vi "PYTHON Get Version and Types__ogtk.vi"(4 "error in (no error)":errorcluster) -> (0 "error out":errorcluster, 2 "types":string[](array[string]), 3 "script server version":string)   [LabVIEW 2012]
doc: "This function returns a version string indicating the Python version implemented in the Python shared library server, (Date and Time when the shared library was created), and [the compiler used to create that shared library]."
uses:
  <userlib>/_OpenG.lib/labpython/lvpython.dll
panel:
  # "PYTHON Get Version and Types.vi\n\nRetrieve the Python shared library version and the supported types\n\nCopyright (C) 2002 Rolf Kalbermatter rolf.kalbermatter@citeng.com\nCopyright (C) 2002 James Kring jim@jimkring.com\n\nPlease visit http://www.OpenG.org to learn about the\nOpen Source LabVIEW software movement.\n\nThis library is free software; you can redistribute it and/or\nmodify it under the terms of the GNU Lesser General Public\nLicense as published by the Free Software Foundation; either\nversion 2.1 of the License, or (at your option) any later version.\nThis library is distributed in the hope that it will be useful,\nbut WITHOUT ANY WARRANTY; without even the implied warranty of\nMERCHANTABILITY or FITNESS FOR A PARTICULAR PURPOSE. See the GNU\nLesser General Public License for more details.\nYou should have received a copy of the GNU Lesser General Public\nLicense along with this library; if not, write to the Free Software\nFoundation, Inc., 59 Temple Place, Suite 330, Boston, MA 02111-1307 USA"
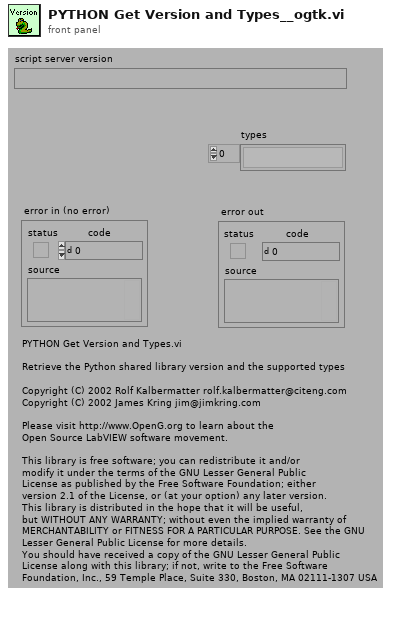
[diagram p1: front panel]
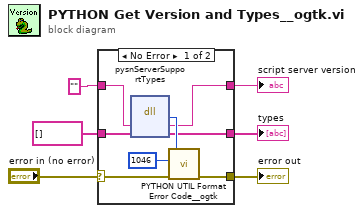
[diagram p0: block diagram]
diagram:
  n1 = case shown="No Error" "error in (no error)" {
    selector: "error in (no error)" -> [w13 w17]
    tunnel: [w10 w15] -> w6
    tunnel: [w12 w17] -> w4
    tunnel: [w9 w16] -> w3
    tunnel: string[] [] ("types") -> [w8 w16]
    tunnel: "" -> [w7 w15]
    frame No Error {
      n2 = dll-call lib="C:/Program Files/National Instruments/LabVIEW 2012/user.lib/_OpenG.lib/labpython/lvpython.*" fn="pysnServerSupportTypes"("version"=w7, "types"=w8) -> (w14:i32, "version"=w10:string, "types"=w9:string[])  [unwired: 3 in, 2 out]
      n3 = call <userlib>:"PYTHON UTIL Format Error Code__ogtk.vi"("error in (no error)"=w13, "code"=1046, "Bool32"=w14) -> ("error out"=w12:errorcluster)  [unwired: 4 in]
    }
    frame Error {
    }
  }
  "error out" <- w4
  "script server version" <- w6
  "types" <- w3
